vi "Default Auto.vi"() -> (3 "Array":T1[](array[typedef]) {"List"."CMDs"."Auto Angle" scale format="%.3f"})   [LabVIEW 2020, in "2023-Auto_CMD.lvlib"]
uses:
  2023-Auto_CMD.lvlib
  Shared Code/TypeDefs/ENUM_Grabber_CMD_Mode Select.ctl
  MotionMaser/ENUM_Pose List.ctl
  MotionMaser/MotionMaster_SubCMD.lvlib
  Shared Code/TypeDefs/Dial_Compase heading unit circle CCW positive.ctl
  ENUM_Drive Mode Select.ctl
  Shared Code/TypeDefs/Cluster_Auto Sequence Settings.ctl
  ENUM_CMD_State.ctl
  Shared Code/TypeDefs/Cluster_Auto Sequence Data.ctl
  Shared Code/TypeDefs/ENUM_AutoSelect.ctl
  Shared Code/TypeDefs/Cluster_AutoSequence.ctl
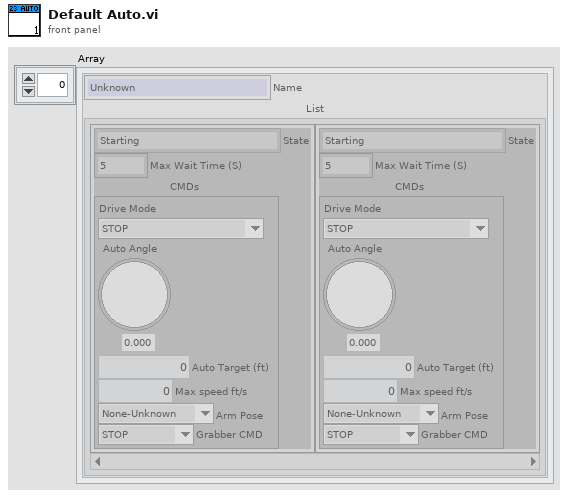
[diagram p1: front panel]
types:
  T1 = typedef "Cluster_AutoSequence.ctl" = cluster{"Name":T2, "List":T3[]}
  T2 = typedef "ENUM_AutoSelect.ctl" = enum16{"Unknown", "Drop High Drive Straight", "Drop mid dock and engage", "Drop High dock and engage", "Auto 4", "Manual"}
  T3 = typedef "Cluster_Auto Sequence Data.ctl" = cluster{"State":T4, "Max Wait Time (S)":dbl, "CMDs":T5}
  T4 = typedef "2023-Auto_CMD.lvlib/ENUM_CMD_State.ctl" = enum16{"Starting", "Idling", "Selecting Sequence", "Selecting Next Step", "Driving to Position", "Stopping", "Grabbing", "Moving Arm", "Rotation Target", "Waiting", "Shutting Down", "Balancing Level", "Configuring"}
  T5 = typedef "Cluster_Auto Sequence Settings.ctl" = cluster{"Drive Mode":T6, "Auto Angle":T7, "Auto Target (ft)":dbl, "Max speed ft/s":dbl, "Arm Pose ":T8, "Grabber CMD":T9}
  T6 = typedef "2023-Auto_CMD.lvlib/ENUM_Drive Mode Select.ctl" = enum16{"STOP", "To Position", "Rotation Absolute", "Balance on Charger"}
  T7 = typedef "Dial_Compase heading unit circle CCW positive.ctl" = dbl
  T8 = typedef "MotionMaster_SubCMD.lvlib/ENUM_Pose List.ctl" = enum16{"None-Unknown", "Intake", "Score High", "Score Mid", "Safe Position", "Home Pos"}
  T9 = typedef "ENUM_Grabber_CMD_Mode Select.ctl" = enum16{"STOP", "Intake", "Eject"}
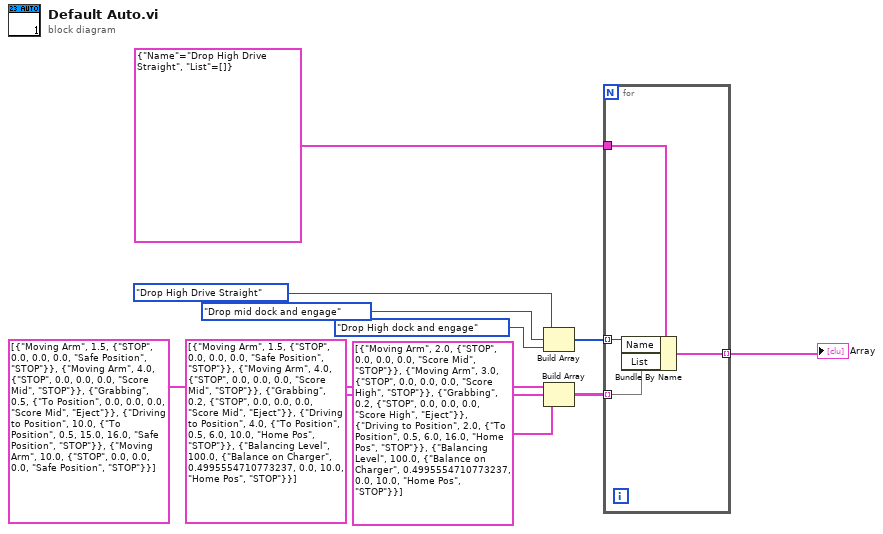
[diagram p0: block diagram]
diagram:
  n1 = Build Array(ENUM_AutoSelect."Drop High Drive Straight" ("CMD Input.Auto Select"), ENUM_AutoSelect."Drop mid dock and engage" ("CMD Input.Auto Select"), ENUM_AutoSelect."Drop High dock and engage" ("CMD Input.Auto Select")) -> (w8:T2[])
  n2 = Build Array(T3[] [{"State"=enum."Moving Arm", "Max Wait Time (S)"=1.5, "CMDs"={"Drive Mode"=enum."STOP", "Auto Angle"=0.0, "Auto Target (ft)"=0.0, "Max speed ft/s"=0.0, "Arm Pose "=enum."Safe Position", "Grabber CMD"=enum."STOP"}}, {"State"=enum."Moving Arm", "Max Wait Time (S)"=4.0, "CMDs"={"Drive Mode"=enum."STOP", "Auto Angle"=0.0, "Auto Target (ft)"=0.0, "Max speed ft/s"=0.0, "Arm Pose "=enum."Score Mid", "Grabber CMD"=enum."STOP"}}, {"State"=enum."Grabbing", "Max Wait Time (S)"=0.5, "CMDs"={"Drive Mode"=enum."To Position", "Auto Angle"=0.0, "Auto Target (ft)"=0.0, "Max speed ft/s"=0.0, "Arm Pose "=enum."Score Mid", "Grabber CMD"=enum."Eject"}}, {"State"=enum."Driving to Position", "Max Wait Time (S)"=10.0, "CMDs"={"Drive Mode"=enum."To Position", "Auto Angle"=0.5, "Auto Target (ft)"=15.0, "Max speed ft/s"=16.0, "Arm Pose "=enum."Safe Position", "Grabber CMD"=enum."STOP"}}, {"State"=enum."Moving Arm", "Max Wait Time (S)"=10.0, "CMDs"={"Drive Mode"=enum."STOP", "Auto Angle"=0.0, "Auto Target (ft)"=0.0, "Max speed ft/s"=0.0, "Arm Pose "=enum."Safe Position", "Grabber CMD"=enum."STOP"}}] ("Drop High Drive Straight"), T3[] [{"State"=enum."Moving Arm", "Max Wait Time (S)"=1.5, "CMDs"={"Drive Mode"=enum."STOP", "Auto Angle"=0.0, "Auto Target (ft)"=0.0, "Max speed ft/s"=0.0, "Arm Pose "=enum."Safe Position", "Grabber CMD"=enum."STOP"}}, {"State"=enum."Moving Arm", "Max Wait Time (S)"=4.0, "CMDs"={"Drive Mode"=enum."STOP", "Auto Angle"=0.0, "Auto Target (ft)"=0.0, "Max speed ft/s"=0.0, "Arm Pose "=enum."Score Mid", "Grabber CMD"=enum."STOP"}}, {"State"=enum."Grabbing", "Max Wait Time (S)"=0.2, "CMDs"={"Drive Mode"=enum."STOP", "Auto Angle"=0.0, "Auto Target (ft)"=0.0, "Max speed ft/s"=0.0, "Arm Pose "=enum."Score Mid", "Grabber CMD"=enum."Eject"}}, {"State"=enum."Driving to Position", "Max Wait Time (S)"=4.0, "CMDs"={"Drive Mode"=enum."To Position", "Auto Angle"=0.5, "Auto Target (ft)"=6.0, "Max speed ft/s"=10.0, "Arm Pose "=enum."Home Pos", "Grabber CMD"=enum."STOP"}}, {"State"=enum."Balancing Level", "Max Wait Time (S)"=100.0, "CMDs"={"Drive Mode"=enum."Balance on Charger", "Auto Angle"=0.4995554710773237, "Auto Target (ft)"=0.0, "Max speed ft/s"=10.0, "Arm Pose "=enum."Home Pos", "Grabber CMD"=enum."STOP"}}] ("Drop mid dock"), T3[] [{"State"=enum."Moving Arm", "Max Wait Time (S)"=2.0, "CMDs"={"Drive Mode"=enum."STOP", "Auto Angle"=0.0, "Auto Target (ft)"=0.0, "Max speed ft/s"=0.0, "Arm Pose "=enum."Score Mid", "Grabber CMD"=enum."STOP"}}, {"State"=enum."Moving Arm", "Max Wait Time (S)"=3.0, "CMDs"={"Drive Mode"=enum."STOP", "Auto Angle"=0.0, "Auto Target (ft)"=0.0, "Max speed ft/s"=0.0, "Arm Pose "=enum."Score High", "Grabber CMD"=enum."STOP"}}, {"State"=enum."Grabbing", "Max Wait Time (S)"=0.2, "CMDs"={"Drive Mode"=enum."STOP", "Auto Angle"=0.0, "Auto Target (ft)"=0.0, "Max speed ft/s"=0.0, "Arm Pose "=enum."Score High", "Grabber CMD"=enum."Eject"}}, {"State"=enum."Driving to Position", "Max Wait Time (S)"=2.0, "CMDs"={"Drive Mode"=enum."To Position", "Auto Angle"=0.5, "Auto Target (ft)"=6.0, "Max speed ft/s"=16.0, "Arm Pose "=enum."Home Pos", "Grabber CMD"=enum."STOP"}}, {"State"=enum."Balancing Level", "Max Wait Time (S)"=100.0, "CMDs"={"Drive Mode"=enum."Balance on Charger", "Auto Angle"=0.4995554710773237, "Auto Target (ft)"=0.0, "Max speed ft/s"=10.0, "Arm Pose "=enum."Home Pos", "Grabber CMD"=enum."STOP"}}] ("Drop High and dock")) -> (w9:T3[][])
  n3 = for {
    tunnel: T1 {"Name"=enum."Drop High Drive Straight", "List"=[]} ("Sequences") -> [w14]
    tunnel: w8 -> [w13] mode=indexing
    tunnel: w9 -> [w12] mode=indexing
    tunnel: [w11] -> w10 mode=indexing
    n4 = Bundle By Name(cluster=w14, "Name"=w13, "List"=w12) -> (w11:T1)
  }
  "Array" <- w10
